vi "Creat Path.vi"(8 "error in (no error)":errorcluster, 11 "base path":path) -> (0 "error out":errorcluster, 3 "output cluster":T1)   [LabVIEW 2014]
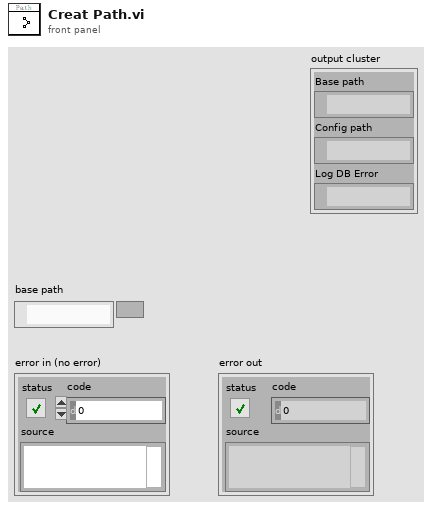
[diagram p1: front panel]
types:
  T1 = cluster{"Base path":path, "Config path":path, "Log DB Error":path}
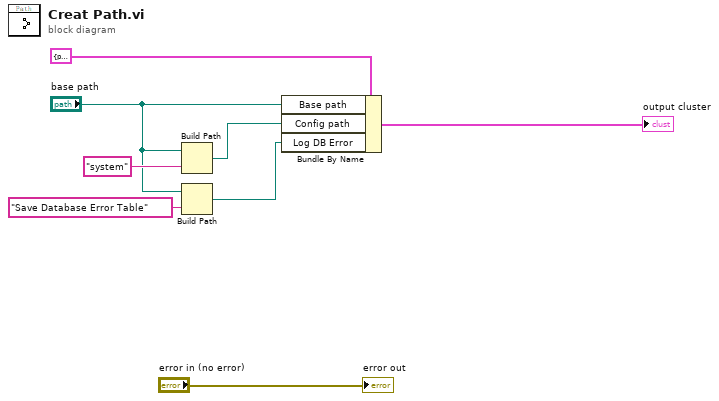
[diagram p0: block diagram]
diagram:
  n1 = Build Path(base path="base path", name or relative path="system") -> (appended path=w4:path)
  n2 = Build Path(base path="base path", name or relative path="Save Database Error Table") -> (appended path=w3:path)
  n3 = Bundle By Name(cluster=T1 {"Base path"=path "", "Config path"=path "", "Log DB Error"=path ""} ("Path"), "Base path"="base path", "Config path"=w4, "Log DB Error"=w3) -> (→"output cluster":T1)
  "error out" <- "error in (no error)"
